vi "Get StationID.vi"(11 "路径":path) -> (3 "Station ID":string)   [LabVIEW 2017]
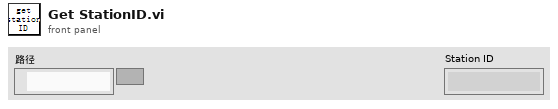
[diagram p1: front panel]
types:
  T1 = enum16{"open", "replace", "create", "open or create", "replace or create", "replace or create with confirmation"}
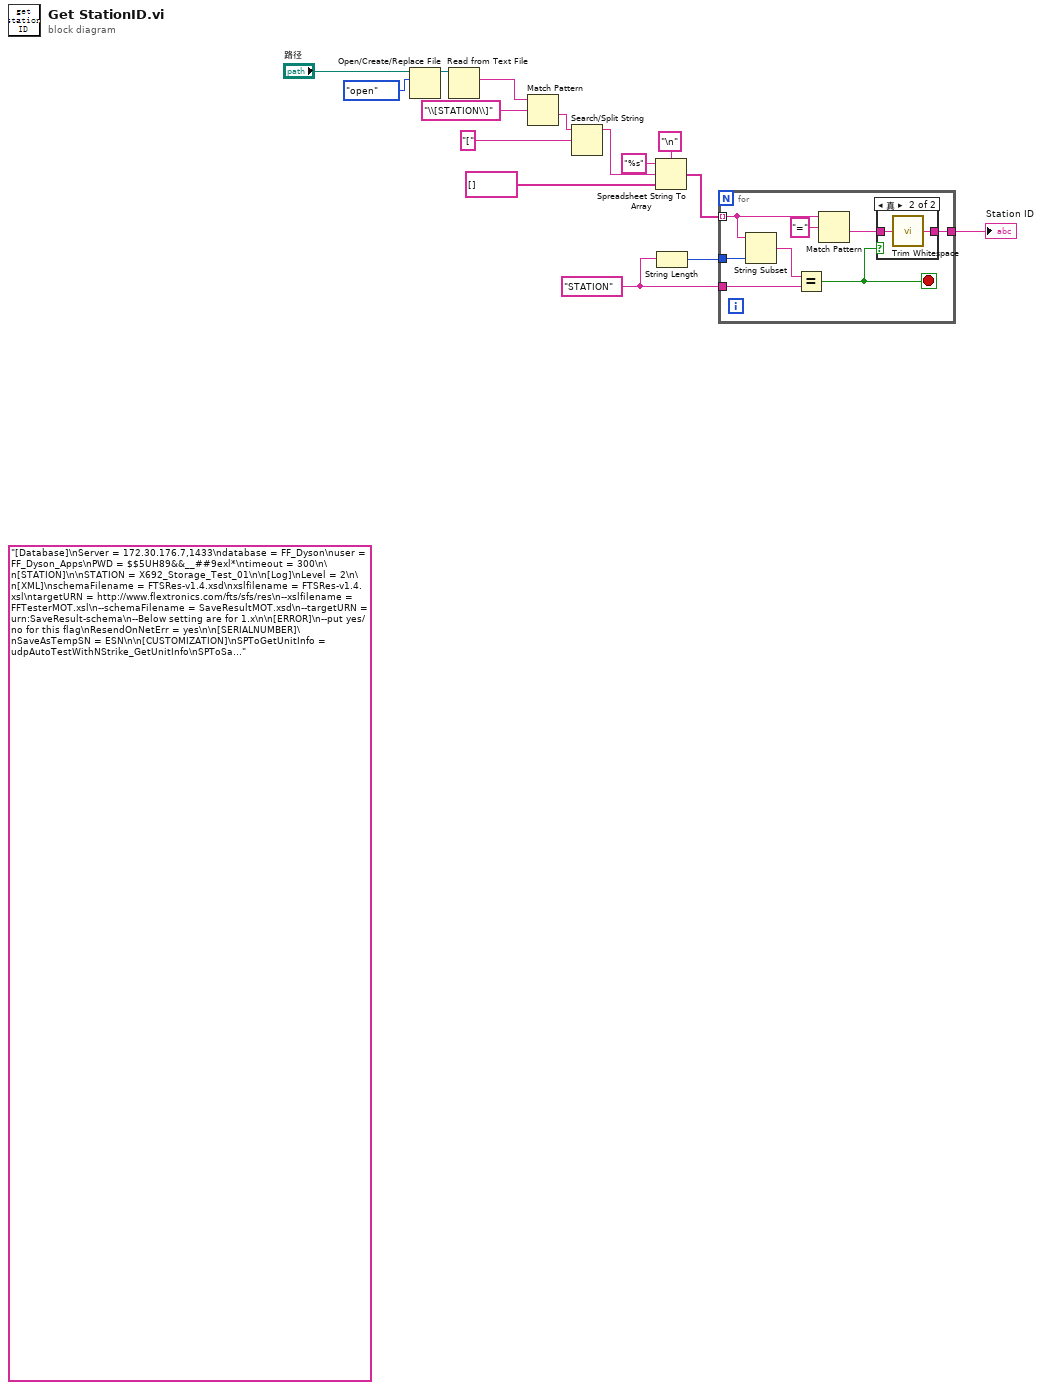
[diagram p0: block diagram]
diagram:
  w2 = "STATION"
  (unwired) "[Database]\nServer = 172.30.176.7,1433\ndatabase = FF_Dyson\nuser = FF_Dyson_Apps\nPWD = $$5UH89&&__##9exl*\ntimeout = 300\n\n[STATION]\n\nSTATION = X692_Storage_Test_01\n\n[Log]\nLevel = 2\n\n[XML]\nschemaFilename = FTSRes-v1.4.xsd\nxslfilename = FTSRes-v1.4.xsl\ntargetURN = http://www.flextronics.com/fts/sfs/res\n--xslfilename = FFTesterMOT.xsl\n--schemaFilename = SaveResultMOT.xsd\n--targetURN = urn:SaveResult-schema\n--Below setting are for 1.x\n\n[ERROR]\n--put yes/no for this flag\nResendOnNetErr = yes\n\n[SERIALNUMBER]\nSaveAsTempSN = ESN\n\n[CUSTOMIZATION]\nSPToGetUnitInfo = udpAutoTestWithNStrike_GetUnitInfo\nSPToSaveTestResult = udpDSN_SaveTestResult\n--SPToSaveTestResult = udpDSN_SaveTestResult_SkipFirstFail\nSPToGetProductStructure = \nSPToGenericFunction = \n\n[GENERICFUNCTIONSMAPPING]\n\n[SaveResultMethod]\nMethod = \n\n[Reporting-DB]\nServer = \ndatabase = \nuser = \nPWD = \n\n"
  n1 = Open/Create/Replace File(file path (use dialog)="路径", operation (0:open)=T1."open" ("操作(0:open)")) -> (refnum out=w13:refnum<file>)  [unwired: 4 in, 2 out]
  n2 = Read from Text File(file (use dialog)=w13) -> (text=w8:string)  [unwired: 3 in, 3 out]
  n3 = Match Pattern(string=w8, regular expression="\\[STATION\\]") -> (after substring=w9:string)  [unwired: 1 in, 3 out]
  n4 = Search/Split String(string=w9, search string/char (-)="[") -> (substring before match=w6:string)  [unwired: 1 in, 2 out]
  n5 = Spreadsheet String To Array(delimiter (Tab)="\n" ("分隔符(Tab)"), format string="%s" ("格式字符串"), spreadsheet string=w6, array type (2D Dbl)=string[] []) -> (array=w3:string[])
  n6 = String Length(string=w2) -> (length=w1:i32)
  n7 = for {
    tunnel: w3 -> [w20] mode=indexing
    tunnel: w2 -> [w21]
    tunnel: w1 -> [w23]
    tunnel: [w16] -> w14
    stop <- w17 stop-if-true
    n8 = String Subset(string=w20, length (rest)=w23) -> (substring=w22:string)  [unwired: 1 in]
    n9 = Equal?(x=w22, y=w21) -> (x = y?=w17:bool)
    n10 = Match Pattern(string=w20, regular expression="=" ("正则表达式")) -> (after substring=w18:string)  [unwired: 1 in, 3 out]
    n11 = case shown="真" w17 {
      tunnel: w18 -> [_ w25]
      tunnel: [_ w24] -> w16
      frame False {
      }
      frame True {
        n12 = call <vilib>:"Trim Whitespace.vi"("string"=w25) -> ("trimmed string"=w24:string)  [unwired: 1 in]
      }
    }
  }
  "Station ID" <- w14
